vi "Test Worry Level.vi"(0 "Test: Divisible By":u64, 1 "LCD":u64, 3 "Worry Level in":u64) -> (2 "Test Result":bool, 5 "Worry Level out":u64)   [LabVIEW 2020, in "AoC 2022.lvlib"]
uses:
  AoC 2022.lvlib
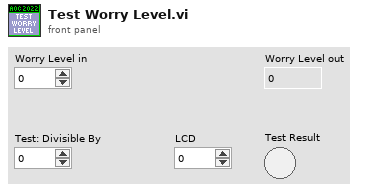
[diagram p1: front panel]
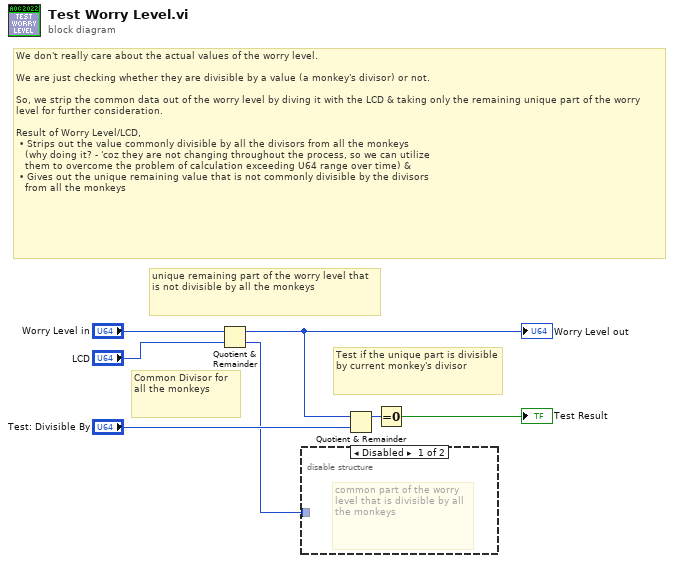
[diagram p0: block diagram]
diagram:
  # "Test if the unique part is divisible by current monkey's divisor"
  # "unique remaining part of the worry level that is not divisible by all the monkeys"
  # "Common Divisor for all the monkeys"
  # "We don't really care about the actual values of the worry level.\n\nWe are just checking whether they are divisible by a value (a monkey's divisor) or not.\n\nSo, we strip the common data out of the worry level by diving it with the LCD & taking only the remaining unique part of the worry level for further consideration.\n\nResult of Worry Level/LCD,\n • Strips out the value commonly divisible by all the divisors from all the monkeys\n   (why doing it? - 'coz they are not changing throughout the process, so we can utilize \n   them to overcome the problem of calculation exceeding U64 range over time) &\n • Gives out the unique remaining value that is not commonly divisible by the divisors\n   from all the monkeys"
  n1 = Quotient & Remainder(x="Worry Level in", y="LCD") -> (x-y*floor(x/y)=w3:u64, floor(x/y)=w1:u64)
  "Worry Level out" <- w3
  n2 = disable-structure shown="Disabled" {
    disable-tunnel: w1 -> [_ _]
    frame Disabled {
      # "common part of the worry level that is divisible by all the monkeys"
    }
    frame Enabled {
    }
  }
  n3 = Quotient & Remainder(x=w3, y="Test: Divisible By") -> (x-y*floor(x/y)=w6:u64)  [unwired: 1 out]
  n4 = Equal To 0?(x=w6) -> (x = 0?=→"Test Result":bool)
